vi "load_array_of_profiles_xml.vi"(8 "error in":errorcluster, 11 "node in":refnum<k20>) -> (0 "error out":errorcluster, 2 "Array of DDS Profiles (8)":T1=[{"Single Tone"={"Frequency [MHz]"=0.0, "Amplitude [dBm]"=0.0, "Phase Offset [rad]"=0.0}, "RAM Mode "=enum."Direct Switch", "Zero-crossing"=FALSE, "No Dwell High"=FALSE, "Function/Static"=FALSE, "RAM Function Settings"=[], "RAM Static Array"=[], "description"=""}], 3 "node":refnum<k20>)   [LabVIEW 2013, in "DDS.lvclass"]
doc: "Load DDS profile from xml. Expected format:\n\n<profile>\n<SingleTone.Frequency units=\"MHz\">%s</SingleTone.Frequency>\n<SingleTone.Amplitude units=\"dBm\">%s</SingleTone.Amplitude>\n<SingleTone.Phase units=\"rad\">%s</SingleTone.Phase>\n<RAMMode>%u</RAMMode>\n<ZeroCrossing>%b</ZeroCrossing>\n<NoDwellHigh>%b</NoDwellHigh>\n<FunctionOrStatic>%b</FunctionOrStatic>\n<RAMFunctionSettings>%s</RAMFunctionSettings>\n<RAMStaticArray>%s</RAMStaticArray>\n</profile>\n\nMTL 2012 Dec 31"
uses:
  DDS.lvclass
  DDS drivers v3/array_of_DDS_profiles.ctl
  DDS drivers v3/DDS_profile.ctl
  DDS drivers v3/DDS RAM mode.ctl
  <vilib>/xml/Close Reference(Node).vi
  <resource>/objmgr/DOMUserDefRef.rc
  <vilib>/xml/NI_XML.lvlib
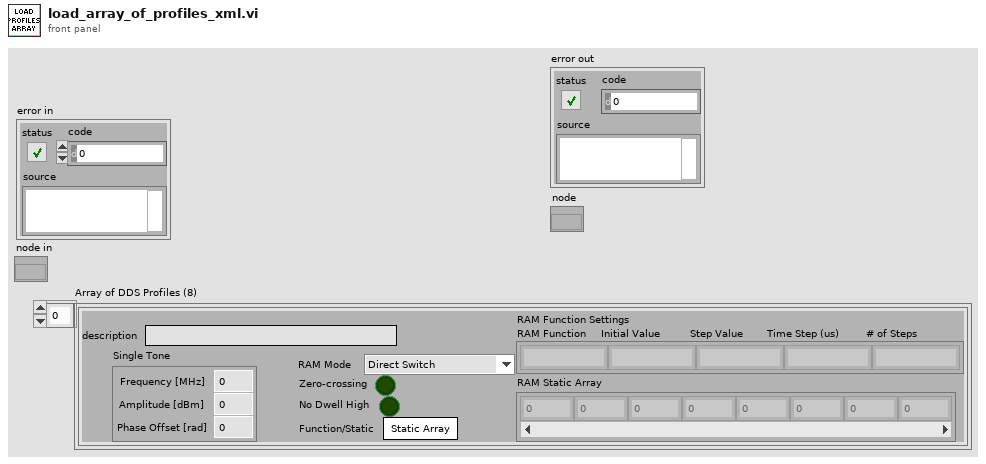
[diagram p1: front panel]
types:
  T1 = typedef "DDS.lvclass/array_of_DDS_profiles.ctl" = T2[]
  T2 = typedef "DDS_profile.ctl" = cluster{"Single Tone":cluster{"Frequency [MHz]":dbl, "Amplitude [dBm]":dbl, "Phase Offset [rad]":dbl}, "RAM Mode ":T3, "Zero-crossing":bool, "No Dwell High":bool, "Function/Static":bool, "RAM Function Settings":string[], "RAM Static Array":dbl[], "description":string}
  T3 = typedef "DDS RAM mode.ctl" = enum16{"Direct Switch", "Ramp Up", "Bidirectional Ramp", "Continuous Bidirectional Ramp", "Continuous Recirculate", "Direct Switch 2", "Direct Switch 3", "Direct Switch 4"}
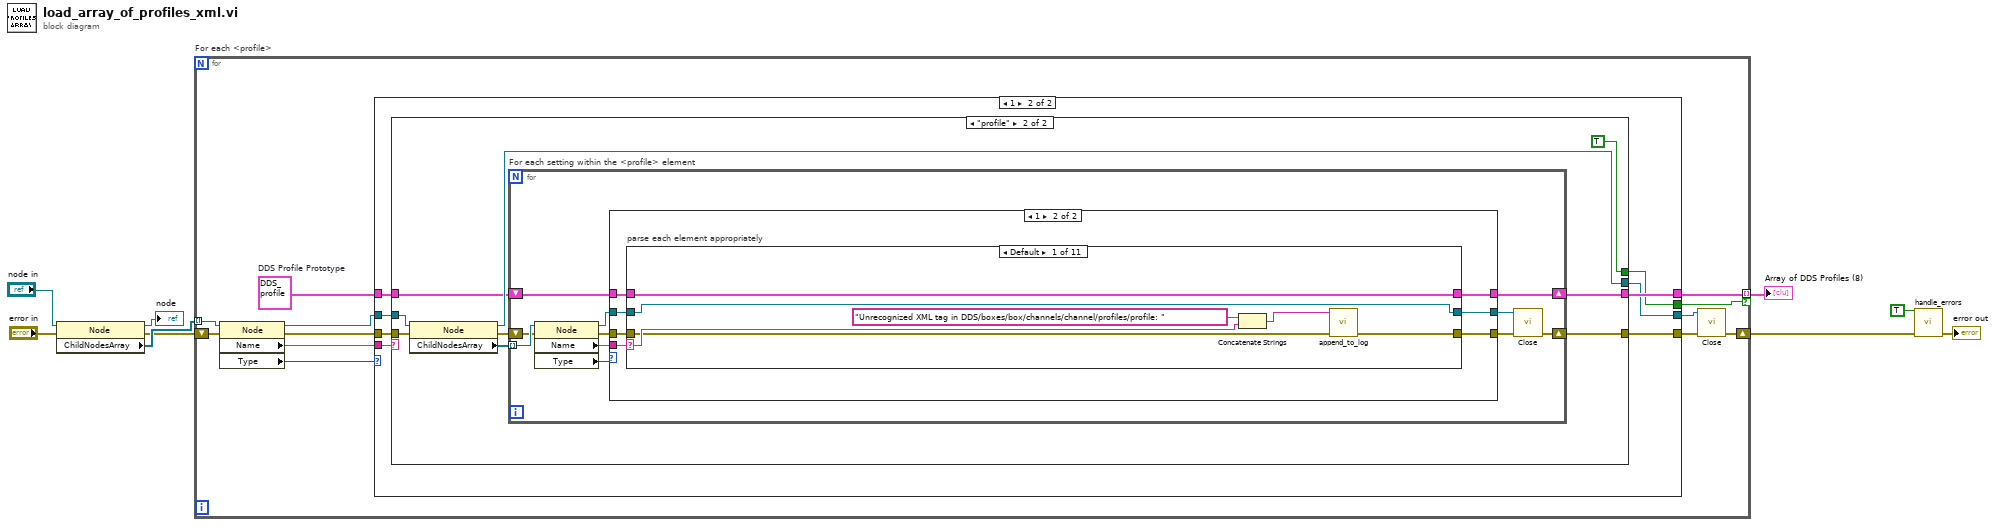
[diagram p0: block diagram]
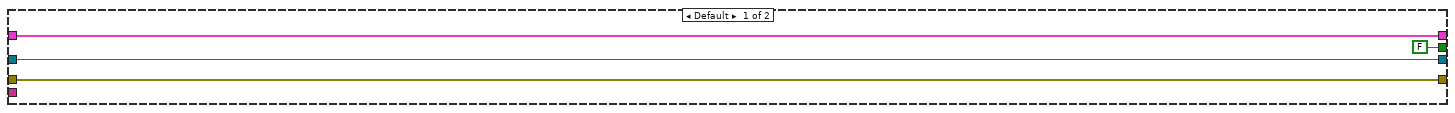
[diagram p2: hidden frame]
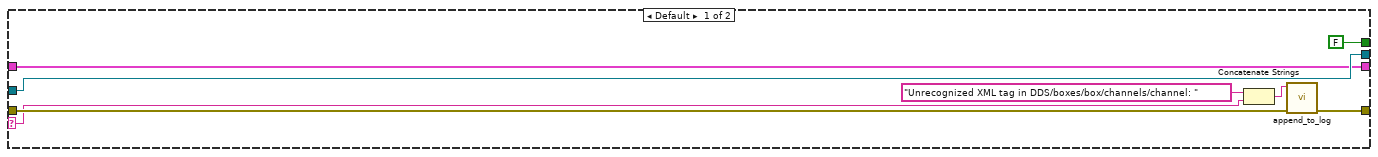
[diagram p3: hidden frame]
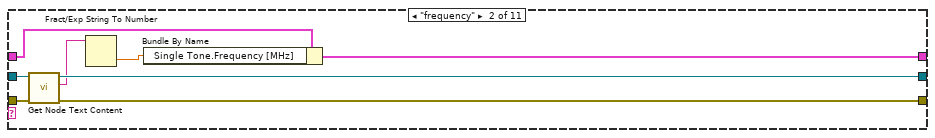
[diagram p5: hidden frame]
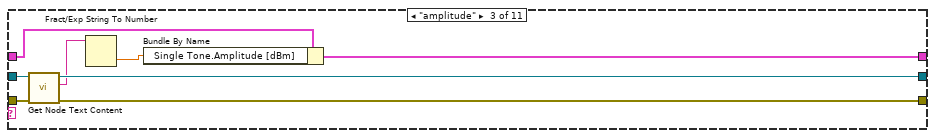
[diagram p6: hidden frame]
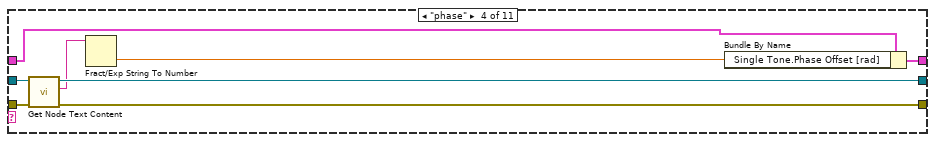
[diagram p7: hidden frame]
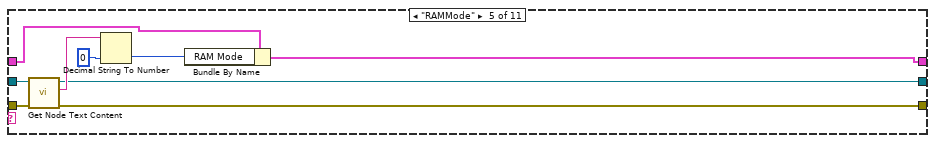
[diagram p8: hidden frame]
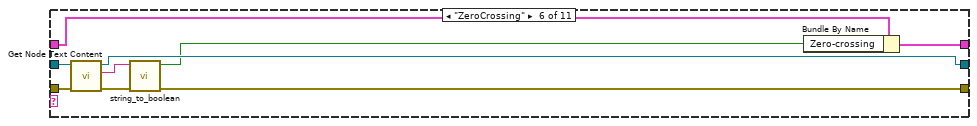
[diagram p9: hidden frame]
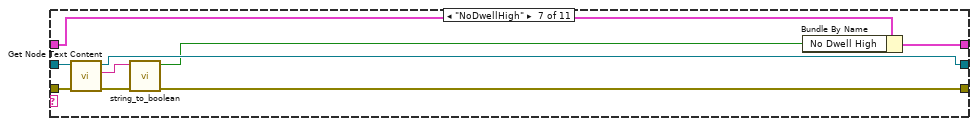
[diagram p10: hidden frame]
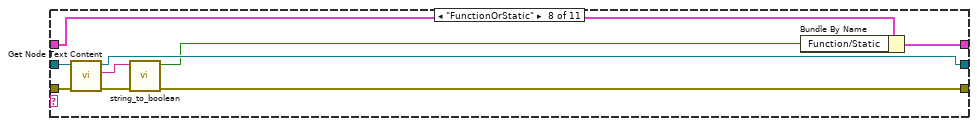
[diagram p11: hidden frame]
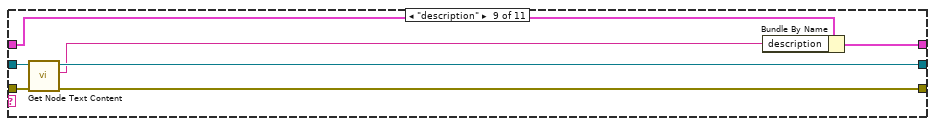
[diagram p12: hidden frame]
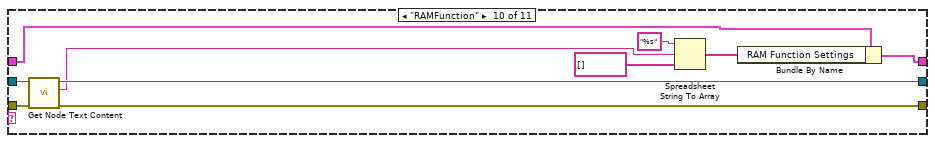
[diagram p13: hidden frame]
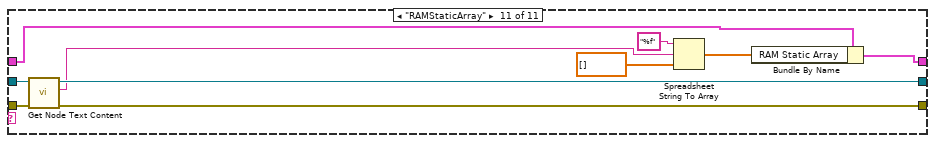
[diagram p14: hidden frame]
diagram:
  n1 = property class="Node"(reference="node in", error in="error in") -> (reference out=→"node":refnum<k20>, error out=w4:errorcluster, "ChildNodesArray"=w6:refnum<k20>[])
  n2 = for "For each <profile>" {
    tunnel: w6 -> [w15] mode=indexing
    shift-right: [w19] -> w3
    shift-left: w4 -> [w17]
    tunnel: [w21] -> w9 mode=indexing if=w10
    w12 = T2 {"Single Tone"={"Frequency [MHz]"=0.0, "Amplitude [dBm]"=0.0, "Phase Offset [rad]"=0.0}, "RAM Mode "=enum."Direct Switch", "Zero-crossing"=FALSE, "No Dwell High"=FALSE, "Function/Static"=FALSE, "RAM Function Settings"=[], "RAM Static Array"=[], "description"=""}  # DDS Profile Prototype
    n3 = property class="Node"(reference=w15, error in=w17) -> (reference out=w14:refnum<k20>, error out=w16:errorcluster, "Name"=w11:string, "Type"=w13:i32)
    n4 = case shown="1" w13 {
      tunnel: [w22 w33] -> w21
      tunnel: [w25 w32] -> w20
      tunnel: w14 -> [w24 w31]
      tunnel: [w24 w30] -> w18
      tunnel: w16 -> [w25 w29]
      tunnel: w12 -> [w22 w28]
      tunnel: w11 -> [_ w27]
      tunnel: [FALSE w26] -> w10
      frame Default {
      }
      frame 1 {
        n5 = case shown="\"profile\"" w27 {
          selector: w27 -> [w36 _]
          tunnel: [w35 w50] -> w33
          tunnel: [w38 w49] -> w32
          tunnel: w31 -> [w37 w48]
          tunnel: [w37 w46] -> w30
          tunnel: w29 -> [w39 w45]
          tunnel: w28 -> [w35 w43]
          tunnel: [FALSE TRUE] -> w26
          frame Default {
            n6 = Concatenate Strings("Unrecognized XML tag in DDS/boxes/box/channels/channel: " ("string"), w36) -> (w40:string)
            n7 = call "append_to_log.vi"("error in"=w39, "string"=w40) -> ("error out"=w38:errorcluster)  [unwired: 9 in]
          }
          frame "profile" {
            n8 = property class="Node"(reference=w48, error in=w45) -> (reference out=w46:refnum<k20>, error out=w44:errorcluster, "ChildNodesArray"=w47:refnum<k20>[])
            n9 = for "For each setting within the <profile> element" {
              tunnel: w47 -> [w61] mode=indexing
              shift-right: [w56] -> w49
              shift-left: w44 -> [w59]
              shift-right: [w54] -> w50
              shift-left: w43 -> [w55]
              n10 = property class="Node"(reference=w61, error in=w59) -> (reference out=w53:refnum<k20>, error out=w58:errorcluster, "Name"=w60:string, "Type"=w51:i32)
              n11 = case shown="1" w51 {
                tunnel: w60 -> [_ w71]
                tunnel: w58 -> [w63 w70]
                tunnel: [w63 w69] -> w57
                tunnel: w55 -> [w64 w68]
                tunnel: [w64 w67] -> w54
                tunnel: w53 -> [w62 w66]
                tunnel: [w62 w65] -> w52
                frame Default {
                }
                frame 1 {
                  n12 = case "parse each element appropriately" shown="Default" w71 {
                    selector: w71 -> [w74 _ _ _ _ _ _ _ _ _ _]
                    tunnel: w70 -> [w73 w84 w92 w98 w106 w117 w126 w136 w143 w151 w164]
                    tunnel: [w72 w83 w91 w97 w105 w114 w124 w131 w139 w148 w158] -> w69
                    tunnel: w68 -> [w78 w82 w94 w102 w111 w120 w121 w134 w141 w155 w163]
                    tunnel: [w78 w81 w89 w101 w110 w119 w127 w138 w145 w154 w162] -> w67
                    tunnel: w66 -> [w77 w86 w93 w100 w104 w118 w129 w137 w144 w153 w165]
                    tunnel: [w77 w85 w90 w99 w103 w116 w128 w135 w142 w152 w161] -> w65
                    frame Default {
                      n13 = Concatenate Strings("Unrecognized XML tag in DDS/boxes/box/channels/channel/profiles/profile: " ("string"), w74) -> (w75:string)
                      n14 = call "append_to_log.vi"("error in"=w73, "string"=w75) -> ("error out"=w72:errorcluster)  [unwired: 9 in]
                    }
                    frame "frequency" {
                      n15 = call <vilib>:"Get Node Text Content.vi"("error in (no error)"=w84, "node in"=w86) -> ("error out"=w83:errorcluster, "node text"=w80:string, "node out"=w85:refnum<k20>)  [unwired: 7 in]
                      n16 = Fract/Exp String To Number(string=w80) -> (number=w79:dbl)  [unwired: 3 in, 1 out]
                      n17 = Bundle By Name(cluster=w82, "Single Tone.Frequency [MHz]"=w79) -> (w81:T2)
                    }
                    frame "amplitude" {
                      n18 = call <vilib>:"Get Node Text Content.vi"("error in (no error)"=w92, "node in"=w93) -> ("error out"=w91:errorcluster, "node text"=w88:string, "node out"=w90:refnum<k20>)  [unwired: 7 in]
                      n19 = Fract/Exp String To Number(string=w88) -> (number=w87:dbl)  [unwired: 3 in, 1 out]
                      n20 = Bundle By Name(cluster=w94, "Single Tone.Amplitude [dBm]"=w87) -> (w89:T2)
                    }
                    frame "phase" {
                      n21 = call <vilib>:"Get Node Text Content.vi"("error in (no error)"=w98, "node in"=w100) -> ("error out"=w97:errorcluster, "node text"=w96:string, "node out"=w99:refnum<k20>)  [unwired: 7 in]
                      n22 = Fract/Exp String To Number(string=w96) -> (number=w95:dbl)  [unwired: 3 in, 1 out]
                      n23 = Bundle By Name(cluster=w102, "Single Tone.Phase Offset [rad]"=w95) -> (w101:T2)
                    }
                    frame "RAMMode" {
                      n24 = call <vilib>:"Get Node Text Content.vi"("error in (no error)"=w106, "node in"=w104) -> ("error out"=w105:errorcluster, "node text"=w109:string, "node out"=w103:refnum<k20>)  [unwired: 7 in]
                      n25 = Decimal String To Number(string=w109, default (0L)=u16 0 ("default (0 I32)")) -> (number=w107:u16)  [unwired: 1 in, 1 out]
                      n26 = Bundle By Name(cluster=w111, "RAM Mode"=w107) -> (w110:T2)
                    }
                    frame "ZeroCrossing" {
                      n27 = call <vilib>:"Get Node Text Content.vi"("error in (no error)"=w117, "node in"=w118) -> ("error out"=w113:errorcluster, "node text"=w115:string, "node out"=w116:refnum<k20>)  [unwired: 7 in]
                      n28 = call "string_to_boolean.vi"("error in"=w113, "string"=w115) -> ("error out"=w114:errorcluster, "boolean"=w112:bool)  [unwired: 8 in]
                      n29 = Bundle By Name(cluster=w120, "Zero-crossing"=w112) -> (w119:T2)
                    }
                    frame "NoDwellHigh" {
                      n30 = call <vilib>:"Get Node Text Content.vi"("error in (no error)"=w126, "node in"=w129) -> ("error out"=w123:errorcluster, "node text"=w125:string, "node out"=w128:refnum<k20>)  [unwired: 7 in]
                      n31 = call "string_to_boolean.vi"("error in"=w123, "string"=w125) -> ("error out"=w124:errorcluster, "boolean"=w122:bool)  [unwired: 8 in]
                      n32 = Bundle By Name(cluster=w121, "No Dwell High"=w122) -> (w127:T2)
                    }
                    frame "FunctionOrStatic" {
                      n33 = call <vilib>:"Get Node Text Content.vi"("error in (no error)"=w136, "node in"=w137) -> ("error out"=w132:errorcluster, "node text"=w133:string, "node out"=w135:refnum<k20>)  [unwired: 7 in]
                      n34 = call "string_to_boolean.vi"("error in"=w132, "string"=w133) -> ("error out"=w131:errorcluster, "boolean"=w130:bool)  [unwired: 8 in]
                      n35 = Bundle By Name(cluster=w134, "Function/Static"=w130) -> (w138:T2)
                    }
                    frame "description" {
                      n36 = call <vilib>:"Get Node Text Content.vi"("error in (no error)"=w143, "node in"=w144) -> ("error out"=w139:errorcluster, "node text"=w140:string, "node out"=w142:refnum<k20>)  [unwired: 7 in]
                      n37 = Bundle By Name(cluster=w141, "description"=w140) -> (w145:T2)
                    }
                    frame "RAMFunction" {
                      n38 = call <vilib>:"Get Node Text Content.vi"("error in (no error)"=w151, "node in"=w153) -> ("error out"=w148:errorcluster, "node text"=w150:string, "node out"=w152:refnum<k20>)  [unwired: 7 in]
                      n39 = Spreadsheet String To Array(format string="%s", spreadsheet string=w150, array type (2D Dbl)=string[] []) -> (array=w146:string[])  [unwired: 1 in]
                      n40 = Bundle By Name(cluster=w155, "RAM Function Settings"=w146) -> (w154:T2)
                    }
                    frame "RAMStaticArray" {
                      n41 = call <vilib>:"Get Node Text Content.vi"("error in (no error)"=w164, "node in"=w165) -> ("error out"=w158:errorcluster, "node text"=w160:string, "node out"=w161:refnum<k20>)  [unwired: 7 in]
                      n42 = Spreadsheet String To Array(format string="%f", spreadsheet string=w160, array type (2D Dbl)=dbl[] []) -> (array=w156:dbl[])  [unwired: 1 in]
                      n43 = Bundle By Name(cluster=w163, "RAM Static Array"=w156) -> (w162:T2)
                    }
                  }
                }
              }
              n44 = call-poly <vilib>:"Close.vi"("error in (no error)"=w57, "node"=w52) -> ("error out"=w56:errorcluster)  [unwired: 7 in]
            }
          }
        }
      }
    }
    n45 = call-poly <vilib>:"Close.vi"("error in (no error)"=w20, "node"=w18) -> ("error out"=w19:errorcluster)  [unwired: 7 in]
  }
  "Array of DDS Profiles (8)" <- w9
  n46 = call "handle_errors.vi"("Exit Operation"=TRUE, "error in (no error)"=w3) -> ("error out"=→"error out":errorcluster)  [unwired: 13 in]
